vi "Set URL Config.vi"(8 "error in (no error)":errorcluster, 10 "url config":T1, 11 "Plugin Model in":refnum<class "Plugin Configuration.lvclass">) -> (0 "error out":errorcluster, 3 "Plugin Model out":refnum<class "Plugin Configuration.lvclass">)   [LabVIEW 2016, in "Plugin Configuration.lvclass"]
uses:
  Plugin Configuration.lvclass
  Typedefs/Plugin Configuration.Typedef.URL Configuration.ctl
  Plugin Configuration.lvclass/Plugin Configuration.ctl
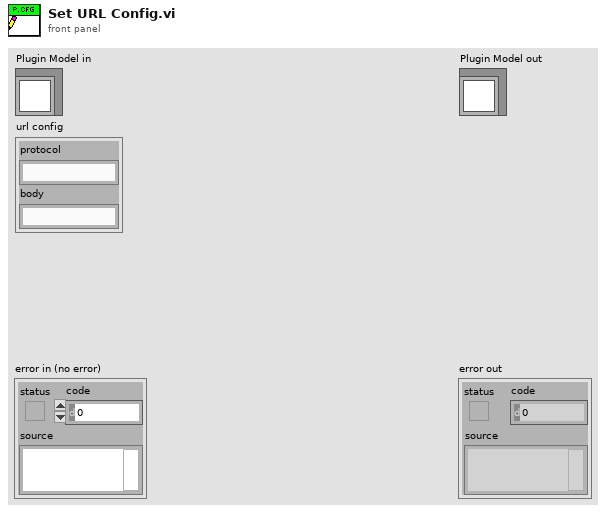
[diagram p1: front panel]
types:
  T1 = typedef "Plugin Configuration.lvclass/Plugin Configuration.Typedef.URL Configuration.ctl" = cluster{"protocol":string, "body":string}
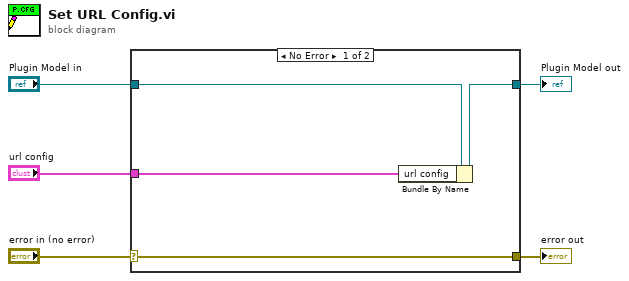
[diagram p0: block diagram]
diagram:
  n1 = case shown="No Error" "error in (no error)" {
    selector: "error in (no error)" -> [w9 w10]
    tunnel: [w9 w10] -> w4
    tunnel: [w7 w11] -> w2
    tunnel: "Plugin Model in" -> [w8 w11]
    tunnel: "url config" -> [w6 _]
    frame No Error {
      n2 = Bundle By Name(cluster=w8, "url config"=w6) -> (w7:refnum<class "Plugin Configuration.lvclass">)
    }
    frame Error {
    }
  }
  "error out" <- w4
  "Plugin Model out" <- w2
